vi "Actuator State Machine.vi"() -> ()   [LabVIEW 2012]
uses:
  Controls/Actuator Shifter.ctl
  <vilib>/Rock Robotics/WPI/Joystick/WPI_JoystickGetSetRefNum.vi
  Globals/Are We Calibrating Actuator.vi
  Globals/Autonomous Tipping.vi
  Globals/Jaguar Commands.vi
  Globals/Max Tipper Angle.vi
panel:
  in  "Actuator Volt Limit":dbl=1.0
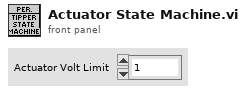
[diagram p1: front panel]
types:
  T1 = typedef "Actuator Shifter.ctl" = enum16{"Wait for Button", "Force Bridge Down", "Hold Bridge Down"}
  T2 = typedef "WPI_JoystickDevRef.ctl" = cluster{"Device":T3}
  T3 = typedef "WPI_JoystickDeviceEnum.ctl" = enum16{"USB 1", "USB 2", "USB 3", "USB 4", "Kinect 1", "Kinect 2"}
  T4 = typedef "WPI_JoystickButtonState.ctl" = cluster{"Button 1":bool, "Button 2":bool, "Button 3":bool, "Button 4":bool, "Button 5":bool, "Button 6":bool, "Button 7":bool, "Button 8":bool, "Button 9":bool, "Button 10":bool, "Button 11":bool, "Button 12":bool}
  T5 = cluster{"axis 1 (x)":dbl, "axis 2 (y)":dbl, "axis 3 (throttle)":dbl, "axis 4":dbl, "axis 5":dbl, "axis 6":dbl}
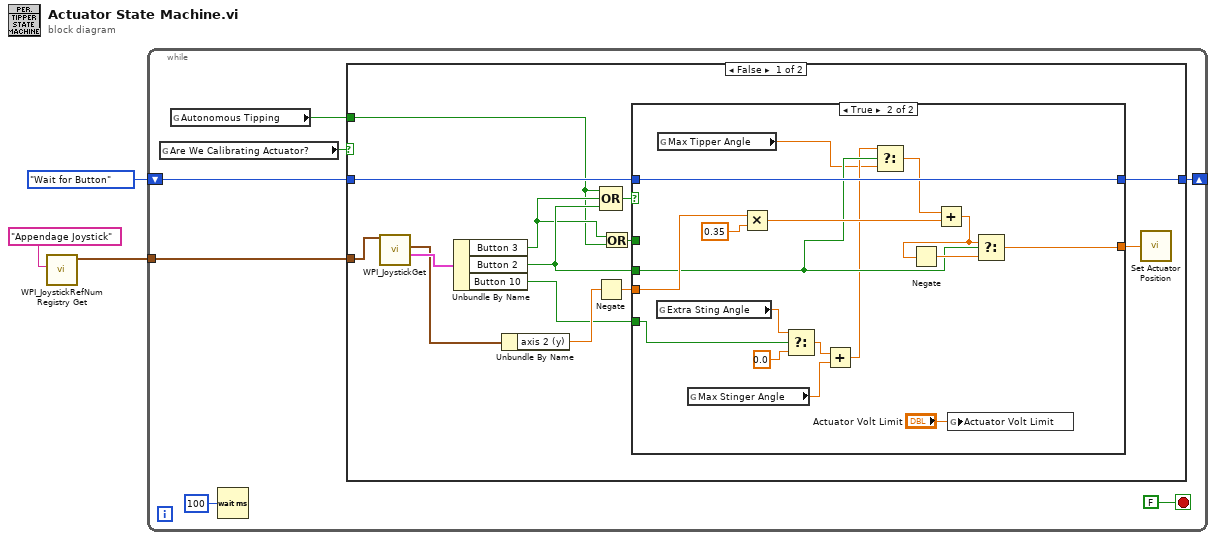
[diagram p0: block diagram]
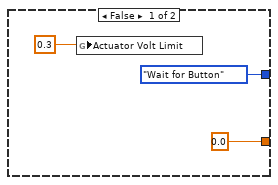
[diagram p2: hidden frame]
diagram:
  n1 = call <vilib>:"WPI_JoystickRefNum Registry Get.vi"("refnum name"="Appendage Joystick") -> ("JoystickDevRef"=w1:T2)  [unwired: 9 in, 1 out]
  n2 = while {
    shift-right: [w7] -> _
    shift-left: Actuator_Shifter."Wait for Button" -> [w6]
    tunnel: w1 -> [w4]
    stop <- FALSE stop-if-true
    n3 = global read "Are We Calibrating Actuator.vi" "Are We Calibrating Actuator?"() -> (w9:bool)
    n4 = global read "Autonomous Tipping.vi" "Autonomous Tipping"() -> (w5:bool)
    n5 = Wait (ms)(milliseconds to wait=u32 100) -> ()  [unwired: 1 out]
    n6 = case shown="False" w9 {
      tunnel: [w23 w45] -> w7
      tunnel: w6 -> [w22 w45]
      tunnel: w5 -> [w17 _]
      tunnel: w4 -> [w14 _]
      frame False {
        n7 = call <vilib>:"WPI_JoystickGet.vi"("JoystickDevRef"=w14) -> ("Buttons"=w24:T4, "Axes"=w16:T5)  [unwired: 4 in, 1 out]
        n8 = Unbundle By Name(w24) -> ("Button 3"=w19:bool, "Button 2"=w20:bool, "Button 10"=w11:bool)
        n9 = Unbundle By Name(w16) -> ("axis 2 (y)"=w15:dbl)
        n10 = Negate(x=w15) -> (-x=w13:dbl)
        n11 = Compound Arithmetic op=OR(w17, w19, w20) -> (w21:bool)
        n12 = Or(x=w19, y=w17) -> (x .or. y?=w18:bool)
        n13 = case shown="True" w21 {
          tunnel: [Actuator_Shifter."Wait for Button" w44] -> w23
          tunnel: w22 -> [_ w44]
          tunnel: w20 -> [_ w30]
          tunnel: w18 -> [_ _]
          tunnel: w13 -> [_ w36]
          tunnel: [0.0 ("Setpoint from Home") w35] -> w12
          tunnel: w11 -> [_ w33]
          frame False {
            n14 = global write "Jaguar Commands.vi" "Actuator Volt Limit"(0.3 ("Actuator Volt Limit")) -> ()
          }
          frame True {
            n15 = global read "Max Tipper Angle.vi" "Extra Sting Angle"() -> (w32:dbl)
            n16 = global read "Max Tipper Angle.vi" "Max Tipper Angle"() -> (w28:dbl)
            n17 = global read "Max Tipper Angle.vi" "Max Stinger Angle"() -> (w38:dbl)
            n18 = Multiply(x=w36, y=0.35) -> (x*y=w39:dbl)
            n19 = Select(t=w32, s=w33, f=0.0) -> (s? t:f=w34:dbl)
            n20 = Add(x=w34, y=w38) -> (x+y=w29:dbl)
            n21 = Select(t=w29, s=w30, f=w28) -> (s? t:f=w37:dbl)
            n22 = Add(x=w37, y=w39) -> (x+y=w41:dbl)
            n23 = Negate(x=w41) -> (-x=w42:dbl)
            n24 = global write "Jaguar Commands.vi" "Actuator Volt Limit"("Actuator Volt Limit") -> ()
            n25 = Select(t=w41, s=w30, f=w42) -> (s? t:f=w35:dbl)
          }
        }
        n26 = call "Set Actuator Position.vi"("Setpoint from Home"=w12) -> ()
      }
      frame True {
      }
    }
  }
